vi "Sync AO and DO.vi"() -> ()   [LabVIEW 2018]
doc: "I. Description:\nThis example demonstrates how to continuously acquire and generate data at the same time, synchronized with one another.\n\nII. Instructions for Running:\n1. Select the physical channel to correspond to where your signal is input on the DAQ device. Also, select the corresponding channel for where your signal is being generated.\n2. Enter the minimum and maximum voltage ranges.\nNote: For better accuracy try to match the input range to the expected voltage level of the measured signal.\n3. Set the sample rate of the acquisition.\nNote: The rate should be at least twice as fast as the maximum frequency component of the signal being acquired. \n6. Select the Rate for the generation\n7. Select what type of signal to generate and the amplitude.\nNote: This example requires two DMA channels to run. If your hardware does not support two DMA channels, you need to set the Data Transfer Mechanism property for the Analog Output Task to use \"Interrupts\". The Data Transfer Mechanism property is located in the DAQmx Channel Property hierarchy at:\n\nDAQmx Channel Property Node>>Analog Output>>General Properties>>Advanced>>Data Transfer and Memory>>Data Transfer Mechanism\n\nRefer to your device documentation to determine how many DMA channels are supported for your hardware.\n\nIII. Block Diagram Steps:\n1. Create an analog input voltage channel. Also, create an analog output voltage channel.\n2. Set the rate for the sample clock. Additionally, define the sample mode to be continuous. Also, set the sample clock rate for the signal generation.\n2a. Call the Get Terminal Name with Device Prefix VI. This will take a Task and a terminal and create a properly formatted device + terminal name to use as the source of the Trigger.\n3. Define the parameters for a Digital Edge Start Trigger. Set the Analog output to trigger off the AI Start Trigger. This is an internal trigger signal.\n4. Use the Basic Function Generator VI to create the signal to be generated.\n5. Call the Start VI to arm the two functions. Make sure the analog output is armed before the analog input. This will ensure both will start at the same time.\n6. Read the waveform data in a loop until the user hits the stop button or an error occurs. The Is Task Done? VI is used to check for errors in the Analog Output Task.\n7. Call the Clear VI to Clear the Task\n8. Use the popup dialog box to display an error if any.\n\nIV. I/O Connections Overview:\nMake sure your signal input/output terminals match the Physical Channel I/O controls."
uses:
  <vilib>/Utility/error.llb/DialogType.ctl
  <vilib>/DAQmx/write.llb/DAQmx Write (Analog Wfm 1Chan NSamp).vi
  <vilib>/DAQmx/write.llb/DAQmx Write (Digital Wfm 1Chan NSamp).vi
  <vilib>/DAQmx/create/channels.llb/DAQmx Create Channel (DO-Digital Output).vi
  <vilib>/DAQmx/create/channels.llb/DAQmx Create Channel (AO-Voltage-Basic).vi
  <vilib>/DAQmx/configure/timing.llb/DAQmx Timing (Sample Clock).vi
  <vilib>/DAQmx/configure/trigger.llb/DAQmx Start Trigger (Digital Edge).vi
  <vilib>/DAQmx/create/channels.llb/DAQmx Create Channel (CO-Pulse Generation-Time).vi
  <vilib>/DAQmx/miscellaneous.llb/DAQmx Fill In Error Info.vi
  <vilib>/Waveform/DWDTOps.llb/DWDT Uncompress Digital.vi
panel:
  out "Waveform Graph":dynamicdata(graph)
  out "Digital Waveform Graph":digitalwaveform(graph)
  in  "rate":dbl=1000.0 caption="Analog Output Update Rate" format="%0.2f"
  in  "minimum value":dbl=-10.0 caption="Output Minimum Value" format="%0.2f"
  in  "maximum value":dbl=10.0 caption="Output Maximum Value" format="%0.2f"
  in  "physical channels":tag="Dev1/ao0" caption="Analog Output Physical Channel"
  in  "Physical Channel":tag="Dev1/port0/line0" caption="Digital Output Physical Channel"
  in  "Rate":dbl=1000.0 caption="Digital Output Update Rate" format="%0.2f"
  in  "stop":bool
  # "For instructions, select Help>>Show Context Help"
  # "Output Channel Parameters"
  # "Timing Parameters"
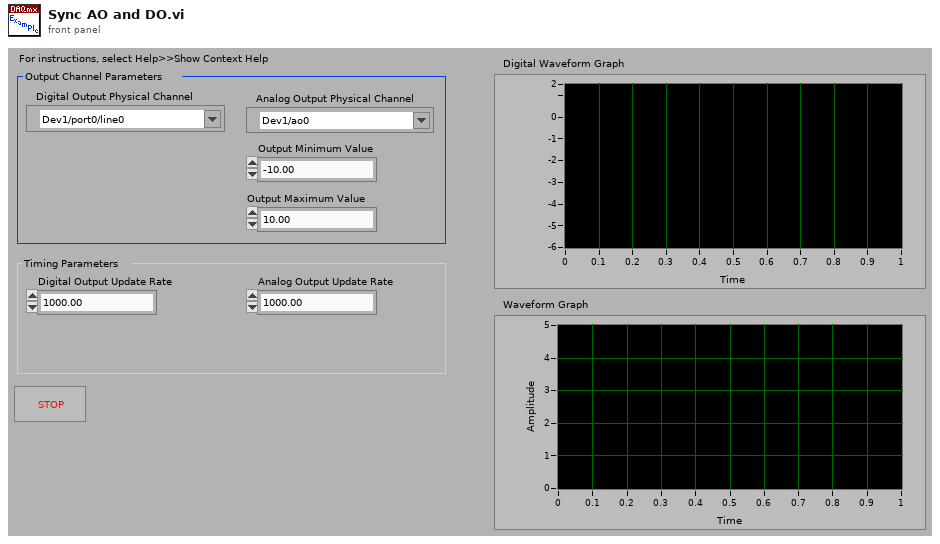
[diagram p1: front panel]
types:
  T1 = typedef "DialogType.ctl" = u16
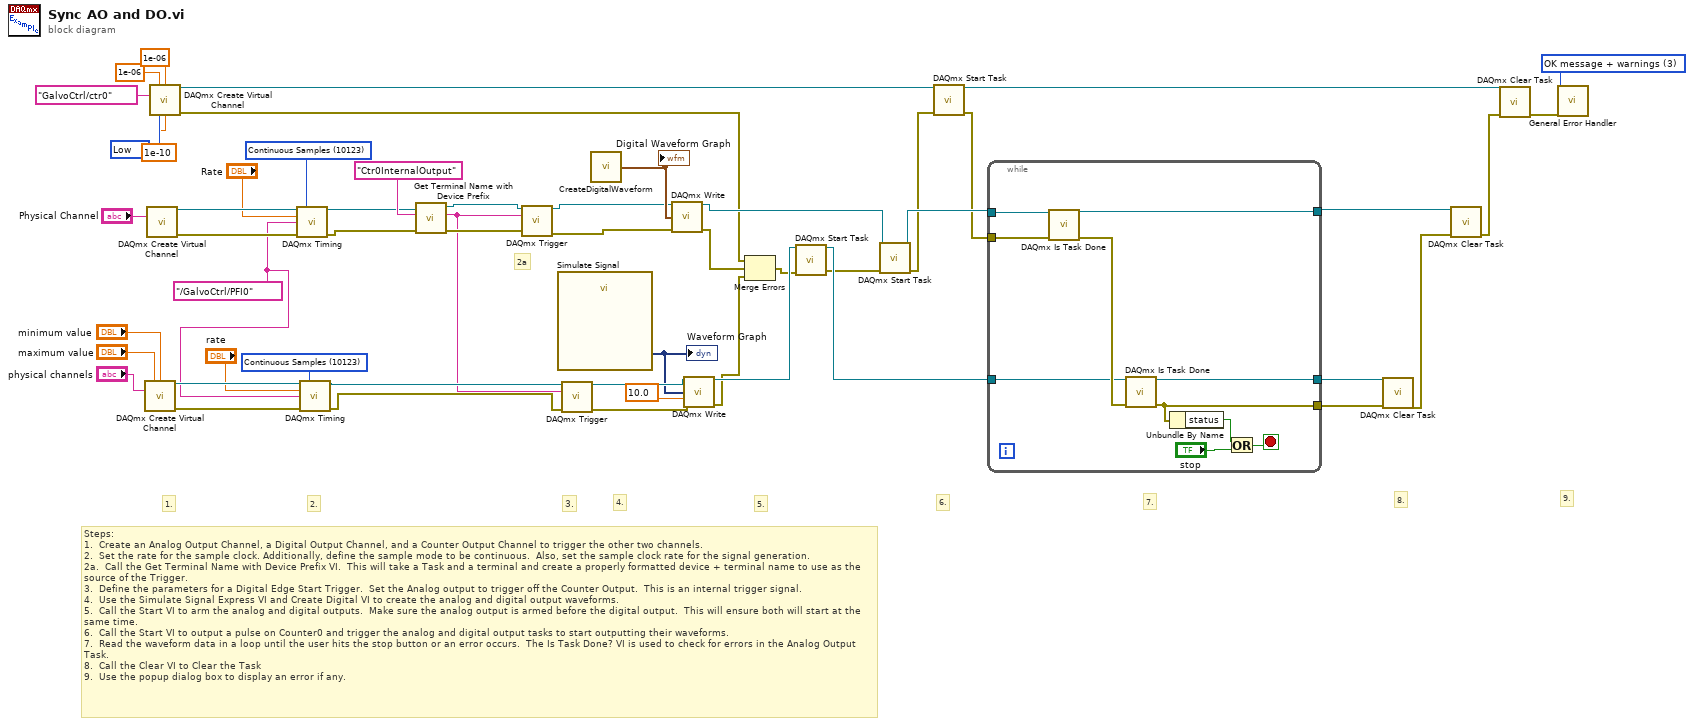
[diagram p0: block diagram]
diagram:
  w26 = 10214 items=["High"=10192, "Low"=10214] ("Idle State")
  w16 = tag "/GalvoCtrl/PFI0" ("source")
  w35 = T1 3 items=["no dialog", "OK message", "continue or stop message", "OK message + warnings", "continue/stop + warnings"] ("type of dialog (OK msg:1)")
  w46 = 10123 items=["Finite Samples"=10178, "Continuous Samples"=10123] ("sample mode")
  w52 = 10123 items=["Finite Samples"=10178, "Continuous Samples"=10123] ("sample mode")
  # "9."
  # "2a"
  # "6."
  # "3."
  # "4."
  # "8."
  # "5."
  # "7."
  # "Steps: \n1.  Create an Analog Output Channel, a Digital Output Channel, and a Counter Output Channel to trigger the other two channels.\n2.  Set the rate for the sample clock. Additionally, define the sample mode to be continuous.  Also, set the sample clock rate for the signal generation.\n2a.  Call the Get Terminal Name with Device Prefix VI.  This will take a Task and a terminal and create a properly formatted device + terminal name to use as the source of the Trigger.\n3.  Define the parameters for a Digital Edge Start Trigger.  Set the Analog output to trigger off the Counter Output.  This is an internal trigger signal.\n4.  Use the Simulate Signal Express VI and Create Digital VI to create the analog and digital output waveforms.\n5.  Call the Start VI to arm the analog and digital outputs.  Make sure the analog output is armed before the digital output.  This will ensure both will start at the same time.\n6.  Call the Start VI to output a pulse on Counter0 and trigger the analog and digital output tasks to start outputting their waveforms.\n7.  Read the waveform data in a loop until the user hits the stop button or an error occurs.  The Is Task Done? VI is used to check for errors in the Analog Output Task.\n8.  Call the Clear VI to Clear the Task\n9.  Use the popup dialog box to display an error if any."
  # "2."
  # "1."
  n1 = call-poly <vilib>:"DAQmx Create Virtual Channel.vi"("maximum value"="maximum value", "minimum value"="minimum value", "physical channels"="physical channels") -> ("task out"=w45:refnum<k21>, "error out"=w44:errorcluster)  [unwired: 6 in, 5 out]
  n2 = call-poly <vilib>:"DAQmx Create Virtual Channel.vi"("lines"="Physical Channel") -> ("task out"=w50:refnum<k21>, "error out"=w51:errorcluster)  [unwired: 6 in, 7 out]
  n3 = call-poly <vilib>:"DAQmx Create Virtual Channel.vi"("high time"=1e-06 ("High Time"), "low time"=1e-06 ("Low Time"), "counter"=tag "GalvoCtrl/ctr0" ("Counter(s)"), "idle state"=w26, "initial delay"=1e-10 ("Initial Delay")) -> ("task out"=w21:refnum<k21>, "error out"=w15:errorcluster)  [unwired: 4 in, 5 out]
  n4 = call-poly <vilib>:"DAQmx Timing.vi"("task/channels in"=w50, "sample mode"=w52, "rate"="Rate", "source"=w16, "error in"=w51) -> ("task out"=w6:refnum<k21>, "error out"=w7:errorcluster)  [unwired: 2 in, 7 out]
  n5 = call-poly <vilib>:"DAQmx Timing.vi"("task/channels in"=w45, "sample mode"=w46, "rate"="rate", "source"=w16, "error in"=w44) -> ("task out"=w8:refnum<k21>, "error out"=w9:errorcluster)  [unwired: 2 in, 7 out]
  n6 = call "Get Terminal Name with Device Prefix.vi"("error in (no error)"=w7, "Local Terminal Name"="Ctr0InternalOutput" ("terminal"), "task/channels in"=w6) -> ("error out"=w5:errorcluster, "Terminal Name with Device Prefix"=w3:tag, "task out"=w2:refnum<k21>)  [unwired: 1 in, 5 out]
  n7 = call-poly <vilib>:"DAQmx Trigger.vi"("task/channels in"=w2, "source"=w3, "error in"=w5) -> ("task out"=w1:refnum<k21>, "error out"=w4:errorcluster)  [unwired: 2 in, 9 out]
  n8 = call "Simulate Signal"() -> ("Triangle"=w28:dynamicdata)  [unwired: 6 in, 9 out]
  "Waveform Graph" <- w28
  n9 = call-poly <vilib>:"DAQmx Trigger.vi"("task/channels in"=w8, "source"=w3, "error in"=w9) -> ("task out"=w37:refnum<k21>, "error out"=w38:errorcluster)  [unwired: 2 in, 9 out]
  n10 = call "CreateDigitalWaveform.vi"() -> ("digital waveform out"=w27:digitalwaveform)
  "Digital Waveform Graph" <- w27
  n11 = call-poly <vilib>:"DAQmx Write.vi"("task/channels in"=w1, "data"=w27, "error in"=w4) -> ("task out"=w29:refnum<k21>, "error out"=w14:errorcluster)  [unwired: 2 in, 9 out]
  n12 = call-poly <vilib>:"DAQmx Write.vi"("task/channels in"=w37, "data"=w28, "timeout"=10.0 ("Wirite Timeout"), "error in"=w38) -> ("task out"=w39:refnum<k21>, "error out"=w13:errorcluster)  [unwired: 1 in, 9 out]
  n13 = Merge Errors(w15, w14, w13) -> (w12:errorcluster)
  n14 = call <vilib>:"DAQmx Start Task.vi"("task/channels in"=w39, "error in"=w12) -> ("task out"=w43:refnum<k21>, "error out"=w11:errorcluster)  [unwired: 12 out]
  n15 = call <vilib>:"DAQmx Start Task.vi"("task/channels in"=w29, "error in"=w11) -> ("task out"=w32:refnum<k21>, "error out"=w10:errorcluster)  [unwired: 12 out]
  n16 = call <vilib>:"DAQmx Start Task.vi"("task/channels in"=w21, "error in"=w10) -> ("task out"=w19:refnum<k21>, "error out"=w20:errorcluster)  [unwired: 12 out]
  n17 = while {
    tunnel: [w63] -> w53
    tunnel: w43 -> [w58]
    tunnel: [w57] -> w42
    tunnel: w32 -> [w56]
    tunnel: w20 -> [w55]
    tunnel: [w54] -> w31
    stop <- w62 stop-if-true
    n18 = call <vilib>:"DAQmx Is Task Done.vi"("task/channels in"=w56, "error in"=w55) -> ("task out"=w63:refnum<k21>, "error out"=w59:errorcluster)  [unwired: 2 in, 10 out]
    n19 = call <vilib>:"DAQmx Is Task Done.vi"("task/channels in"=w58, "error in"=w59) -> ("task out"=w57:refnum<k21>, "error out"=w54:errorcluster)  [unwired: 12 out]
    n20 = Unbundle By Name(w54) -> ("status"=w60:bool)
    n21 = Or(x=w60, y="stop") -> (x .or. y?=w62:bool)
  }
  n22 = call <vilib>:"DAQmx Clear Task.vi"("task in"=w42, "error in"=w31) -> ("error out"=w30:errorcluster)  [unwired: 13 out]
  n23 = call <vilib>:"DAQmx Clear Task.vi"("task in"=w53, "error in"=w30) -> ("error out"=w18:errorcluster)  [unwired: 13 out]
  n24 = call <vilib>:"DAQmx Clear Task.vi"("task in"=w19, "error in"=w18) -> ("error out"=w17:errorcluster)  [unwired: 13 out]
  n25 = call <vilib>:"General Error Handler.vi"("type of dialog (OK msg:1)"=w35, "error in (no error)"=w17) -> ()  [unwired: 1 in, 13 out]
